vi "Begin.vi"(8 "error in":errorcluster) -> (0 "error out":errorcluster)   [LabVIEW 2019]
doc: "Called before other user functions, this VI is expected to open initial I/O refnums, load in file data, and do all program initialization. Notice that the <B>error out</B> terminal is simply used for data flow. Wiring it to other structures or subVIs ensures that this VI runs first."
uses:
  <vilib>/Rock Robotics/WPI/DriverStation/WPI_DriverStationRobotMode2.ctl
  <vilib>/Rock Robotics/WPI/Joystick/WPI_JoystickDeviceEnum.ctl
  <vilib>/Rock Robotics/WPI/ThirdParty/Phoenix-LabVIEW/Motor Controller/Controls/CTRE_Phoenix_MotorControl_NeutralMode.ctl
  <vilib>/Rock Robotics/WPI/Solenoid/WPI_SolenoidChannel.ctl
  <vilib>/Rock Robotics/SystemInterfaces/DIO/FPGA_DIOChannel.ctl
  Robot Global Data.vi
  <vilib>/Rock Robotics/WPI/Utilities/WPI_GetSetVariantRefNum.vi
  <vilib>/Rock Robotics/WPI/Solenoid/WPI_SolenoidOpenDouble.vi
  <vilib>/Rock Robotics/WPI/ThirdParty/REV Robotics/SPARK MAX/Typedef/Spark MAX Idle Mode.ctl
  <vilib>/Rock Robotics/WPI/ThirdParty/Phoenix-LabVIEW/Motor Controller/Controls/CTRE_Phoenix_MotorControl_SupplyCurrentLimitConfiguration.ctl
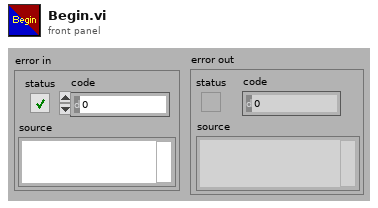
[diagram p1: front panel]
types:
  T1 = typedef "WPI_JoystickDeviceEnum.ctl" = enum16{"USB 0", "USB 1", "USB 2", "USB 3", "USB 4", "USB 5"}
  T2 = typedef "WPI_DriverStationRobotMode2.ctl" = enum16{"Autonomous Disabled", "Autonomous Enabled", "Teleop Disabled", "Teleop Enabled", "Disconnected", "Finish", "Test Disabled", "Test Enabled", "Emergency Stopped"}
  T3 = typedef "WPI_JoystickDevRef.ctl" = cluster{"Device":T1}
  T4 = typedef "Spark MAX Idle Mode.ctl" = enum16{"Coast", "Brake"}
  T5 = typedef "WPI_MotorControlDeviceRef.ctl" = cluster{"DeviceStatus":errorcluster, "Type":T6, "PWM":cluster{"PWM Channel":T7, "DeadBand":T8}, "CAN":cluster{"Device Number":u8, "SetOutput VI Ref":variant, "GetOutput VI Ref":variant, "Enable VI Ref":variant, "Disable VI Ref":variant, "Data":variant}, "Invert":bool, "DIO PWM":cluster{"PWM \"Enable\" Channel":T7, "DIOChannel":T9, "PWM Rate":dbl}}
  T6 = typedef "WPI_MotorControlType.ctl" = enum16{"PWM", "CAN", "DIO PWM"}
  T7 = typedef "FPGA_DIOPWMChannel.ctl" = enum8{"PWM 0", "PWM 1", "PWM 2", "PWM 3", "PWM 4", "PWM 5", "PWM 6", "PWM 7", "PWM 8", "PWM 9", "PWM MXP 0", "PWM MXP 1", "PWM MXP 2", "PWM MXP 3", "PWM MXP 4", "PWM MXP 5", "PWM MXP 6", "PWM MXP 7", "PWM MXP 8", "PWM MXP 9", "Invalid"}
  T8 = typedef "WPI_PWMDeadband.ctl" = cluster{"Name":string, "maxPositivePwm":i32, "minPositivePwm":i32, "centerPwm":i32, "maxNegativePwm":i32, "minNegativePwm":i32, "angularRange":u16}
  T9 = typedef "FPGA_DIOChannel.ctl" = enum8{"DIO 0", "DIO 1", "DIO 2", "DIO 3", "DIO 4", "DIO 5", "DIO 6", "DIO 7", "DIO 8", "DIO 9", "DIO MXP 0", "DIO MXP 1", "DIO MXP 2", "DIO MXP 3", "DIO MXP 4", "DIO MXP 5", "DIO MXP 6", "DIO MXP 7", "DIO MXP 8", "DIO MXP 9", "DIO MXP 10", "DIO MXP 11", "DIO MXP 12", "DIO MXP 13", "DIO MXP 14", "DIO MXP 15", "SPI Port CS1", "SPI Port CS2", "SPI Port CS3", "SPI Port MISO", "SPI Port MOSI", "Invalid"}
  T10 = typedef "CTRE_Phoenix_MotorControl_NeutralMode.ctl" = enum8{"EEPROMSetting", "Override to Coast", "Override to Brake"}
  T11 = typedef "CTRE_Phoenix_MotorControl_SupplyCurrentLimitConfiguration.ctl" = cluster{"Enable?":bool, "Current Limit":dbl, "Threshold Current":dbl, "Threshold Time":dbl}
  T12 = typedef "WPI_SolenoidChannel.ctl" = enum8{"Solenoid 0", "Solenoid 1", "Solenoid 2", "Solenoid 3", "Solenoid 4", "Solenoid 5", "Solenoid 6", "Solenoid 7", "Invalid"}
  T13 = typedef "WPI_CompressorDevRef.ctl" = cluster{"DevStatus":errorcluster, "Pneumatics Control Module":u8}
  T14 = typedef "WPI_SolenoidDevRef.ctl" = cluster{"DevStatus":errorcluster, "Pneumatics Control Module":u8, "Forward Solenoid Channel":T12, "Reverse Solenoid Channel":T12}
  T15 = typedef "WPI_DigitalInputDevRef.ctl" = cluster{"DevStatus":errorcluster, "DIO Channel":T9}
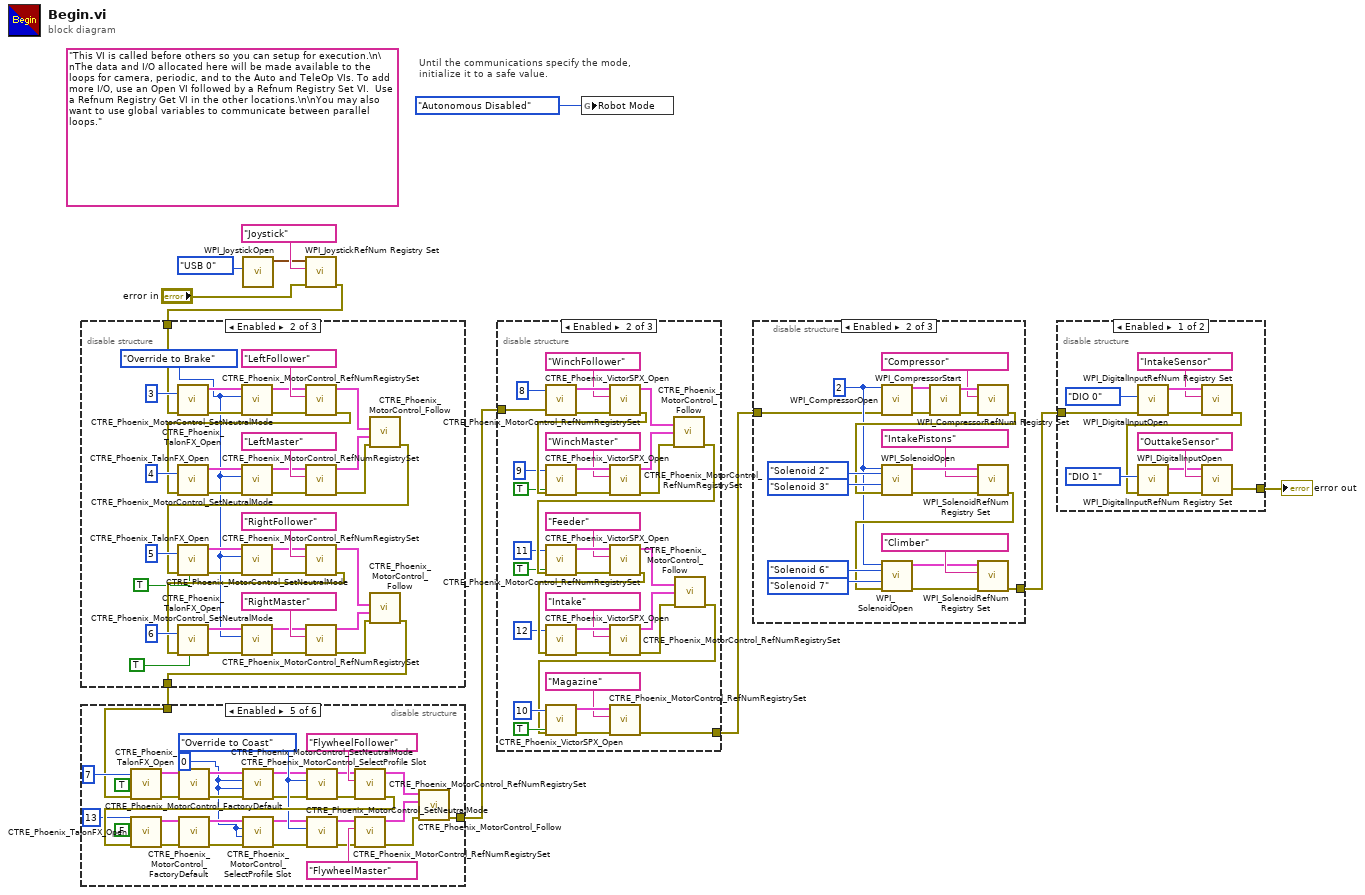
[diagram p0: block diagram]
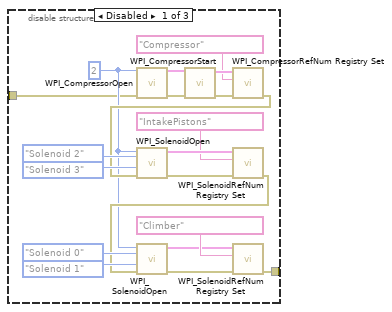
[diagram p3: hidden frame]
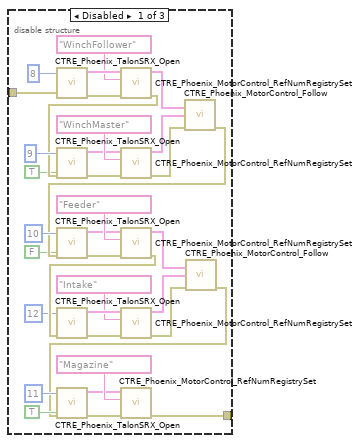
[diagram p5: hidden frame]
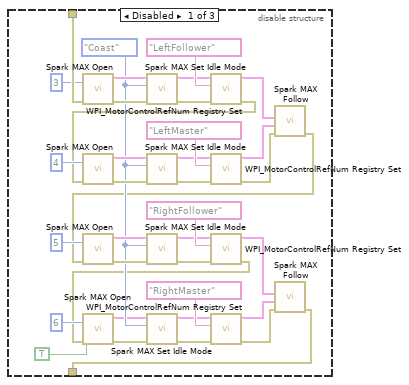
[diagram p7: hidden frame]
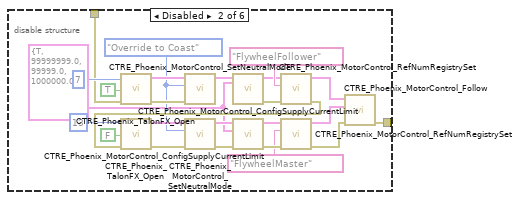
[diagram p10: hidden frame]
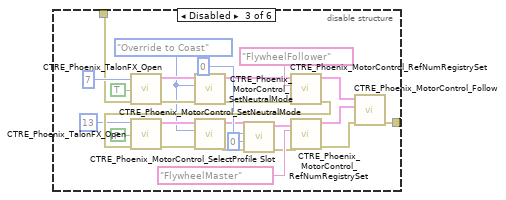
[diagram p11: hidden frame]
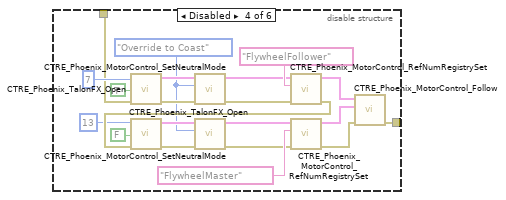
[diagram p12: hidden frame]
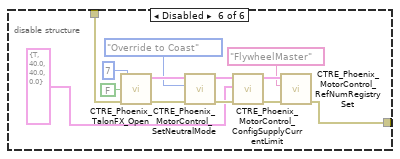
[diagram p13: hidden frame]
diagram:
  (unwired) "This VI is called before others so you can setup for execution.\n\nThe data and I/O allocated here will be made available to the loops for camera, periodic, and to the Auto and TeleOp VIs. To add more I/O, use an Open VI followed by a Refnum Registry Set VI.  Use a Refnum Registry Get VI in the other locations.\n\nYou may also want to use global variables to communicate between parallel loops."
  # "Until the communications specify the mode,\ninitialize it to a safe value."
  n1 = call <vilib>:"WPI_JoystickOpen.vi"("JoystickDevice"=WPI_JoystickDeviceEnum."USB 0") -> ("JoystickDevRef"=w9:T3)  [unwired: 10 in]
  n2 = call <vilib>:"WPI_JoystickRefNum Registry Set.vi"("error in (no error)"="error in", "refnum name"="Joystick", "JoystickDevRef"=w9) -> ("error out"=w7:errorcluster)  [unwired: 7 in, 1 out]
  n3 = disable-structure shown="Enabled" {
    disable-tunnel: w7 -> [w48 w52 w87]
    disable-tunnel: [w47 w51 w87] -> w5
    frame Disabled {
      w22 = Spark_MAX_Idle_Mode."Coast" ("Idle Mode")
      n4 = call <vilib>:"Spark MAX Open.vi"("error in (no error)"=w48, "Device Number"=u8 3) -> ("error out"=w33:errorcluster, "MotorControlDeviceRef"=w34:T5)  [unwired: 8 in]
      n5 = call <vilib>:"Spark MAX Set Idle Mode.vi"("error in (no error)"=w33, "Idle Mode"=w22, "MotorControlDeviceRef in"=w34) -> ("error out"=w31:errorcluster, "MotorControlDeviceRef out"=w32:T5)  [unwired: 7 in]
      n6 = call <vilib>:"WPI_MotorControlRefNum Registry Set.vi"("error in (no error)"=w31, "refnum name"="LeftFollower", "MotorControlDevRef"=w32) -> ("error out"=w17:errorcluster, "MotorControlDevRef"=w38:T5)  [unwired: 7 in]
      n7 = call <vilib>:"Spark MAX Open.vi"("error in (no error)"=w17, "Device Number"=u8 4) -> ("error out"=w29:errorcluster, "MotorControlDeviceRef"=w30:T5)  [unwired: 8 in]
      n8 = call <vilib>:"Spark MAX Set Idle Mode.vi"("error in (no error)"=w29, "Idle Mode"=w22, "MotorControlDeviceRef in"=w30) -> ("error out"=w27:errorcluster, "MotorControlDeviceRef out"=w28:T5)  [unwired: 7 in]
      n9 = call <vilib>:"WPI_MotorControlRefNum Registry Set.vi"("error in (no error)"=w27, "refnum name"="LeftMaster", "MotorControlDevRef"=w28) -> ("error out"=w16:errorcluster, "MotorControlDevRef"=w37:T5)  [unwired: 7 in]
      n10 = call <vilib>:"Spark MAX Follow.vi"("error in (no error)"=w16, "Master Controller"=w37, "MotorControlDeviceRef"=w38) -> ("error out"=w15:errorcluster)  [unwired: 7 in, 1 out]
      n11 = call <vilib>:"Spark MAX Open.vi"("error in (no error)"=w15, "Device Number"=u8 5) -> ("error out"=w25:errorcluster, "MotorControlDeviceRef"=w26:T5)  [unwired: 8 in]
      n12 = call <vilib>:"Spark MAX Set Idle Mode.vi"("error in (no error)"=w25, "Idle Mode"=w22, "MotorControlDeviceRef in"=w26) -> ("error out"=w23:errorcluster, "MotorControlDeviceRef out"=w24:T5)  [unwired: 7 in]
      n13 = call <vilib>:"WPI_MotorControlRefNum Registry Set.vi"("error in (no error)"=w23, "refnum name"="RightFollower", "MotorControlDevRef"=w24) -> ("error out"=w14:errorcluster, "MotorControlDevRef"=w36:T5)  [unwired: 7 in]
      n14 = call <vilib>:"Spark MAX Open.vi"("error in (no error)"=w14, "Invert"=TRUE, "Device Number"=u8 6) -> ("error out"=w20:errorcluster, "MotorControlDeviceRef"=w21:T5)  [unwired: 7 in]
      n15 = call <vilib>:"Spark MAX Set Idle Mode.vi"("error in (no error)"=w20, "Idle Mode"=w22, "MotorControlDeviceRef in"=w21) -> ("error out"=w18:errorcluster, "MotorControlDeviceRef out"=w19:T5)  [unwired: 7 in]
      n16 = call <vilib>:"WPI_MotorControlRefNum Registry Set.vi"("error in (no error)"=w18, "refnum name"="RightMaster", "MotorControlDevRef"=w19) -> ("error out"=w13:errorcluster, "MotorControlDevRef"=w35:T5)  [unwired: 7 in]
      n17 = call <vilib>:"Spark MAX Follow.vi"("error in (no error)"=w13, "Master Controller"=w35, "MotorControlDeviceRef"=w36) -> ("error out"=w47:errorcluster)  [unwired: 7 in, 1 out]
    }
    frame Enabled {
      w50 = CTRE_Phoenix_MotorControl_NeutralMode."Override to Brake" ("Motor Control Neutral Mode")
      n18 = call <vilib>:"CTRE_Phoenix_TalonFX_Open.vi"("error in"=w52, "Device Number"=u8 3) -> ("error out"=w73:errorcluster, "CAN Talon SRX Ref"=w74:T5)  [unwired: 8 in]
      n19 = call <vilib>:"CTRE_Phoenix_MotorControl_SetNeutralMode.vi"("error in (no error)"=w73, "Motor Control Neutral Mode"=w50, "PhoenixMotorControlDevRef"=w74) -> ("error out"=w71:errorcluster, "PhoenixMotorControlDevRef"=w72:T5)  [unwired: 7 in]
      n20 = call <vilib>:"CTRE_Phoenix_MotorControl_RefNumRegistrySet.vi"("error in (no error)"=w71, "refnum name"="LeftFollower", "PhoenixMotorControlDevRef"=w72) -> ("error out"=w58:errorcluster, "PhoenixMotorControlDevRef"=w78:T5)  [unwired: 7 in]
      n21 = call <vilib>:"CTRE_Phoenix_TalonFX_Open.vi"("error in"=w58, "Device Number"=u8 4) -> ("error out"=w69:errorcluster, "CAN Talon SRX Ref"=w70:T5)  [unwired: 8 in]
      n22 = call <vilib>:"CTRE_Phoenix_MotorControl_SetNeutralMode.vi"("error in (no error)"=w69, "Motor Control Neutral Mode"=w50, "PhoenixMotorControlDevRef"=w70) -> ("error out"=w67:errorcluster, "PhoenixMotorControlDevRef"=w68:T5)  [unwired: 7 in]
      n23 = call <vilib>:"CTRE_Phoenix_MotorControl_RefNumRegistrySet.vi"("error in (no error)"=w67, "refnum name"="LeftMaster", "PhoenixMotorControlDevRef"=w68) -> ("error out"=w57:errorcluster, "PhoenixMotorControlDevRef"=w77:T5)  [unwired: 7 in]
      n24 = call <vilib>:"CTRE_Phoenix_MotorControl_Follow.vi"("error in (no error)"=w57, "Master Controller to Follow"=w77, "PhoenixMotorControlDevRef"=w78) -> ("error out"=w56:errorcluster)  [unwired: 7 in, 1 out]
      n25 = call <vilib>:"CTRE_Phoenix_TalonFX_Open.vi"("Invert"=TRUE, "error in"=w56, "Device Number"=u8 5) -> ("error out"=w65:errorcluster, "CAN Talon SRX Ref"=w66:T5)  [unwired: 7 in]
      n26 = call <vilib>:"CTRE_Phoenix_MotorControl_SetNeutralMode.vi"("error in (no error)"=w65, "Motor Control Neutral Mode"=w50, "PhoenixMotorControlDevRef"=w66) -> ("error out"=w63:errorcluster, "PhoenixMotorControlDevRef"=w64:T5)  [unwired: 7 in]
      n27 = call <vilib>:"CTRE_Phoenix_MotorControl_RefNumRegistrySet.vi"("error in (no error)"=w63, "refnum name"="RightFollower", "PhoenixMotorControlDevRef"=w64) -> ("error out"=w55:errorcluster, "PhoenixMotorControlDevRef"=w76:T5)  [unwired: 7 in]
      n28 = call <vilib>:"CTRE_Phoenix_TalonFX_Open.vi"("Invert"=TRUE, "error in"=w55, "Device Number"=u8 6) -> ("error out"=w61:errorcluster, "CAN Talon SRX Ref"=w62:T5)  [unwired: 7 in]
      n29 = call <vilib>:"CTRE_Phoenix_MotorControl_SetNeutralMode.vi"("error in (no error)"=w61, "Motor Control Neutral Mode"=w50, "PhoenixMotorControlDevRef"=w62) -> ("error out"=w59:errorcluster, "PhoenixMotorControlDevRef"=w60:T5)  [unwired: 7 in]
      n30 = call <vilib>:"CTRE_Phoenix_MotorControl_RefNumRegistrySet.vi"("error in (no error)"=w59, "refnum name"="RightMaster", "PhoenixMotorControlDevRef"=w60) -> ("error out"=w54:errorcluster, "PhoenixMotorControlDevRef"=w75:T5)  [unwired: 7 in]
      n31 = call <vilib>:"CTRE_Phoenix_MotorControl_Follow.vi"("error in (no error)"=w54, "Master Controller to Follow"=w75, "PhoenixMotorControlDevRef"=w76) -> ("error out"=w51:errorcluster)  [unwired: 7 in, 1 out]
    }
    frame Disabled {
    }
  }
  n32 = disable-structure shown="Enabled" {
    disable-tunnel: w5 -> [w88 w109 w134 w155 w187 w193]
    disable-tunnel: [w88 w89 w122 w143 w177 w190] -> w4
    frame Disabled {
    }
    frame Disabled {
      w97 = T11 {"Enable?"=TRUE, "Current Limit"=99999999.0, "Threshold Current"=99999.0, "Threshold Time"=1000000.0} ("Supply Current Limit Configuration")
      w98 = CTRE_Phoenix_MotorControl_NeutralMode."Override to Coast" ("Motor Control Neutral Mode")
      n33 = call <vilib>:"CTRE_Phoenix_TalonFX_Open.vi"("Invert"=TRUE, "error in"=w109, "Device Number"=u8 7) -> ("error out"=w110:errorcluster, "CAN Talon SRX Ref"=w111:T5)  [unwired: 7 in]
      n34 = call <vilib>:"CTRE_Phoenix_MotorControl_SetNeutralMode.vi"("error in (no error)"=w110, "Motor Control Neutral Mode"=w98, "PhoenixMotorControlDevRef"=w111) -> ("PhoenixMotorControlDevRef"=w106:T5)  [unwired: 7 in, 1 out]
      n35 = call <vilib>:"CTRE_Phoenix_MotorControl_ConfigSupplyCurrentLimit.vi"("Supply Current Limit Configuration"=w97, "PhoenixMotorControlDevRef"=w106) -> ("error out"=w108:errorcluster, "PhoenixMotorControlDevRef"=w107:T5)  [unwired: 8 in]
      n36 = call <vilib>:"CTRE_Phoenix_MotorControl_RefNumRegistrySet.vi"("error in (no error)"=w108, "refnum name"="FlywheelFollower", "PhoenixMotorControlDevRef"=w107) -> ("error out"=w99:errorcluster, "PhoenixMotorControlDevRef"=w95:T5)  [unwired: 7 in]
      n37 = call <vilib>:"CTRE_Phoenix_TalonFX_Open.vi"("Invert"=FALSE, "error in"=w99, "Device Number"=u8 13) -> ("error out"=w104:errorcluster, "CAN Talon SRX Ref"=w105:T5)  [unwired: 7 in]
      n38 = call <vilib>:"CTRE_Phoenix_MotorControl_SetNeutralMode.vi"("error in (no error)"=w104, "Motor Control Neutral Mode"=w98, "PhoenixMotorControlDevRef"=w105) -> ("error out"=w100:errorcluster, "PhoenixMotorControlDevRef"=w101:T5)  [unwired: 7 in]
      n39 = call <vilib>:"CTRE_Phoenix_MotorControl_ConfigSupplyCurrentLimit.vi"("error in (no error)"=w100, "Supply Current Limit Configuration"=w97, "PhoenixMotorControlDevRef"=w101) -> ("error out"=w103:errorcluster, "PhoenixMotorControlDevRef"=w102:T5)  [unwired: 7 in]
      n40 = call <vilib>:"CTRE_Phoenix_MotorControl_RefNumRegistrySet.vi"("error in (no error)"=w103, "refnum name"="FlywheelMaster", "PhoenixMotorControlDevRef"=w102) -> ("error out"=w93:errorcluster, "PhoenixMotorControlDevRef"=w94:T5)  [unwired: 7 in]
      n41 = call <vilib>:"CTRE_Phoenix_MotorControl_Follow.vi"("error in (no error)"=w93, "Master Controller to Follow"=w94, "PhoenixMotorControlDevRef"=w95) -> ("error out"=w89:errorcluster)  [unwired: 7 in, 1 out]
    }
    frame Disabled {
      w130 = CTRE_Phoenix_MotorControl_NeutralMode."Override to Coast" ("Motor Control Neutral Mode")
      n42 = call <vilib>:"CTRE_Phoenix_TalonFX_Open.vi"("Invert"=TRUE, "error in"=w134, "Device Number"=u8 7) -> ("error out"=w135:errorcluster, "CAN Talon SRX Ref"=w136:T5)  [unwired: 7 in]
      n43 = call <vilib>:"CTRE_Phoenix_MotorControl_SetNeutralMode.vi"("error in (no error)"=w135, "Motor Control Neutral Mode"=w130, "PhoenixMotorControlDevRef"=w136) -> ("error out"=w115:errorcluster, "PhoenixMotorControlDevRef"=w116:T5)  [unwired: 7 in]
      n44 = call <vilib>:"CTRE_Phoenix_MotorControl_RefNumRegistrySet.vi"("error in (no error)"=w115, "refnum name"="FlywheelFollower", "PhoenixMotorControlDevRef"=w116) -> ("error out"=w131:errorcluster, "PhoenixMotorControlDevRef"=w128:T5)  [unwired: 7 in]
      n45 = call <vilib>:"CTRE_Phoenix_TalonFX_Open.vi"("Invert"=FALSE, "error in"=w131, "Device Number"=u8 13) -> ("error out"=w132:errorcluster, "CAN Talon SRX Ref"=w133:T5)  [unwired: 7 in]
      n46 = call <vilib>:"CTRE_Phoenix_MotorControl_SetNeutralMode.vi"("error in (no error)"=w132, "Motor Control Neutral Mode"=w130, "PhoenixMotorControlDevRef"=w133) -> ("error out"=w117:errorcluster, "PhoenixMotorControlDevRef"=w118:T5)  [unwired: 7 in]
      n47 = call <vilib>:"CTRE_Phoenix_MotorControl_SelectProfile Slot.vi"("error in (no error)"=w117, "pidLoopIdx"=0, "slotIdx"=0, "PhoenixMotorControlDevRef"=w118) -> ("error out"=w120:errorcluster, "PhoenixMotorControlDevRef"=w121:T5)  [unwired: 6 in]
      n48 = call <vilib>:"CTRE_Phoenix_MotorControl_RefNumRegistrySet.vi"("error in (no error)"=w120, "refnum name"="FlywheelMaster", "PhoenixMotorControlDevRef"=w121) -> ("error out"=w126:errorcluster, "PhoenixMotorControlDevRef"=w127:T5)  [unwired: 7 in]
      n49 = call <vilib>:"CTRE_Phoenix_MotorControl_Follow.vi"("error in (no error)"=w126, "Master Controller to Follow"=w127, "PhoenixMotorControlDevRef"=w128) -> ("error out"=w122:errorcluster)  [unwired: 7 in, 1 out]
    }
    frame Disabled {
      w151 = CTRE_Phoenix_MotorControl_NeutralMode."Override to Coast" ("Motor Control Neutral Mode")
      n50 = call <vilib>:"CTRE_Phoenix_TalonFX_Open.vi"("Invert"=TRUE, "error in"=w155, "Device Number"=u8 7) -> ("error out"=w156:errorcluster, "CAN Talon SRX Ref"=w157:T5)  [unwired: 7 in]
      n51 = call <vilib>:"CTRE_Phoenix_MotorControl_SetNeutralMode.vi"("error in (no error)"=w156, "Motor Control Neutral Mode"=w151, "PhoenixMotorControlDevRef"=w157) -> ("error out"=w142:errorcluster, "PhoenixMotorControlDevRef"=w141:T5)  [unwired: 7 in]
      n52 = call <vilib>:"CTRE_Phoenix_MotorControl_RefNumRegistrySet.vi"("error in (no error)"=w142, "refnum name"="FlywheelFollower", "PhoenixMotorControlDevRef"=w141) -> ("error out"=w152:errorcluster, "PhoenixMotorControlDevRef"=w149:T5)  [unwired: 7 in]
      n53 = call <vilib>:"CTRE_Phoenix_TalonFX_Open.vi"("Invert"=FALSE, "error in"=w152, "Device Number"=u8 13) -> ("error out"=w153:errorcluster, "CAN Talon SRX Ref"=w154:T5)  [unwired: 7 in]
      n54 = call <vilib>:"CTRE_Phoenix_MotorControl_SetNeutralMode.vi"("error in (no error)"=w153, "Motor Control Neutral Mode"=w151, "PhoenixMotorControlDevRef"=w154) -> ("error out"=w139:errorcluster, "PhoenixMotorControlDevRef"=w140:T5)  [unwired: 7 in]
      n55 = call <vilib>:"CTRE_Phoenix_MotorControl_RefNumRegistrySet.vi"("error in (no error)"=w139, "refnum name"="FlywheelMaster", "PhoenixMotorControlDevRef"=w140) -> ("error out"=w147:errorcluster, "PhoenixMotorControlDevRef"=w148:T5)  [unwired: 7 in]
      n56 = call <vilib>:"CTRE_Phoenix_MotorControl_Follow.vi"("error in (no error)"=w147, "Master Controller to Follow"=w148, "PhoenixMotorControlDevRef"=w149) -> ("error out"=w143:errorcluster)  [unwired: 7 in, 1 out]
    }
    frame Enabled {
      w164 = 0 ("slotIdx")
      w185 = CTRE_Phoenix_MotorControl_NeutralMode."Override to Coast" ("Motor Control Neutral Mode")
      n57 = call <vilib>:"CTRE_Phoenix_TalonFX_Open.vi"("Invert"=TRUE, "error in"=w187, "Device Number"=u8 7) -> ("error out"=w169:errorcluster, "CAN Talon SRX Ref"=w170:T5)  [unwired: 7 in]
      n58 = call <vilib>:"CTRE_Phoenix_MotorControl_FactoryDefault.vi"("error in"=w169, "PhoenixMotorControlDevRef"=w170) -> ("error out"=w168:errorcluster, "PhoenixMotorControlDevRef"=w167:T5)  [unwired: 8 in]
      n59 = call <vilib>:"CTRE_Phoenix_MotorControl_SelectProfile Slot.vi"("error in (no error)"=w168, "pidLoopIdx"=w164, "slotIdx"=w164, "PhoenixMotorControlDevRef"=w167) -> ("error out"=w162:errorcluster, "PhoenixMotorControlDevRef"=w163:T5)  [unwired: 6 in]
      n60 = call <vilib>:"CTRE_Phoenix_MotorControl_SetNeutralMode.vi"("error in (no error)"=w162, "Motor Control Neutral Mode"=w185, "PhoenixMotorControlDevRef"=w163) -> ("error out"=w175:errorcluster, "PhoenixMotorControlDevRef"=w176:T5)  [unwired: 7 in]
      n61 = call <vilib>:"CTRE_Phoenix_MotorControl_RefNumRegistrySet.vi"("error in (no error)"=w175, "refnum name"="FlywheelFollower", "PhoenixMotorControlDevRef"=w176) -> ("error out"=w186:errorcluster, "PhoenixMotorControlDevRef"=w183:T5)  [unwired: 7 in]
      n62 = call <vilib>:"CTRE_Phoenix_TalonFX_Open.vi"("Invert"=FALSE, "error in"=w186, "Device Number"=u8 13) -> ("error out"=w171:errorcluster, "CAN Talon SRX Ref"=w172:T5)  [unwired: 7 in]
      n63 = call <vilib>:"CTRE_Phoenix_MotorControl_FactoryDefault.vi"("error in"=w171, "PhoenixMotorControlDevRef"=w172) -> ("error out"=w165:errorcluster, "PhoenixMotorControlDevRef"=w166:T5)  [unwired: 8 in]
      n64 = call <vilib>:"CTRE_Phoenix_MotorControl_SelectProfile Slot.vi"("error in (no error)"=w165, "pidLoopIdx"=w164, "slotIdx"=w164, "PhoenixMotorControlDevRef"=w166) -> ("error out"=w160:errorcluster, "PhoenixMotorControlDevRef"=w161:T5)  [unwired: 6 in]
      n65 = call <vilib>:"CTRE_Phoenix_MotorControl_SetNeutralMode.vi"("error in (no error)"=w160, "Motor Control Neutral Mode"=w185, "PhoenixMotorControlDevRef"=w161) -> ("error out"=w173:errorcluster, "PhoenixMotorControlDevRef"=w174:T5)  [unwired: 7 in]
      n66 = call <vilib>:"CTRE_Phoenix_MotorControl_RefNumRegistrySet.vi"("error in (no error)"=w173, "refnum name"="FlywheelMaster", "PhoenixMotorControlDevRef"=w174) -> ("error out"=w181:errorcluster, "PhoenixMotorControlDevRef"=w182:T5)  [unwired: 7 in]
      n67 = call <vilib>:"CTRE_Phoenix_MotorControl_Follow.vi"("error in (no error)"=w181, "Master Controller to Follow"=w182, "PhoenixMotorControlDevRef"=w183) -> ("error out"=w177:errorcluster)  [unwired: 7 in, 1 out]
    }
    frame Disabled {
      n68 = call <vilib>:"CTRE_Phoenix_TalonFX_Open.vi"("Invert"=FALSE, "error in"=w193, "Device Number"=u8 7) -> ("error out"=w199:errorcluster, "CAN Talon SRX Ref"=w198:T5)  [unwired: 7 in]
      n69 = call <vilib>:"CTRE_Phoenix_MotorControl_SetNeutralMode.vi"("error in (no error)"=w199, "Motor Control Neutral Mode"=CTRE_Phoenix_MotorControl_NeutralMode."Override to Coast", "PhoenixMotorControlDevRef"=w198) -> ("error out"=w192:errorcluster, "PhoenixMotorControlDevRef"=w202:T5)  [unwired: 7 in]
      n70 = call <vilib>:"CTRE_Phoenix_MotorControl_ConfigSupplyCurrentLimit.vi"("error in (no error)"=w192, "Supply Current Limit Configuration"=T11 {"Enable?"=TRUE, "Current Limit"=40.0, "Threshold Current"=40.0, "Threshold Time"=0.0}, "PhoenixMotorControlDevRef"=w202) -> ("error out"=w200:errorcluster, "PhoenixMotorControlDevRef"=w201:T5)  [unwired: 7 in]
      n71 = call <vilib>:"CTRE_Phoenix_MotorControl_RefNumRegistrySet.vi"("error in (no error)"=w200, "refnum name"="FlywheelMaster", "PhoenixMotorControlDevRef"=w201) -> ("error out"=w190:errorcluster)  [unwired: 7 in, 1 out]
    }
  }
  n72 = disable-structure shown="Enabled" {
    disable-tunnel: w4 -> [w208 w243 w273]
    disable-tunnel: [w207 w242 w273] -> w3
    frame Disabled {
      n73 = call <vilib>:"CTRE_Phoenix_TalonSRX_Open.vi"("error in"=w208, "Device Number"=u8 8) -> ("error out"=w220:errorcluster, "CAN Talon SRX Ref"=w221:T5)  [unwired: 8 in]
      n74 = call <vilib>:"CTRE_Phoenix_MotorControl_RefNumRegistrySet.vi"("error in (no error)"=w220, "refnum name"="WinchFollower", "PhoenixMotorControlDevRef"=w221) -> ("error out"=w213:errorcluster, "PhoenixMotorControlDevRef"=w209:T5)  [unwired: 7 in]
      n75 = call <vilib>:"CTRE_Phoenix_TalonSRX_Open.vi"("Invert"=TRUE, "error in"=w213, "Device Number"=u8 9) -> ("error out"=w215:errorcluster, "CAN Talon SRX Ref"=w214:T5)  [unwired: 7 in]
      n76 = call <vilib>:"CTRE_Phoenix_MotorControl_RefNumRegistrySet.vi"("error in (no error)"=w215, "refnum name"="WinchMaster", "PhoenixMotorControlDevRef"=w214) -> ("error out"=w211:errorcluster, "PhoenixMotorControlDevRef"=w210:T5)  [unwired: 7 in]
      n77 = call <vilib>:"CTRE_Phoenix_MotorControl_Follow.vi"("error in (no error)"=w211, "Master Controller to Follow"=w210, "PhoenixMotorControlDevRef"=w209) -> ("error out"=w224:errorcluster)  [unwired: 7 in, 1 out]
      n78 = call <vilib>:"CTRE_Phoenix_TalonSRX_Open.vi"("Invert"=FALSE, "error in"=w224, "Device Number"=u8 10) -> ("error out"=w230:errorcluster, "CAN Talon SRX Ref"=w229:T5)  [unwired: 7 in]
      n79 = call <vilib>:"CTRE_Phoenix_MotorControl_RefNumRegistrySet.vi"("error in (no error)"=w230, "refnum name"="Feeder", "PhoenixMotorControlDevRef"=w229) -> ("error out"=w237:errorcluster, "PhoenixMotorControlDevRef"=w206:T5)  [unwired: 7 in]
      n80 = call <vilib>:"CTRE_Phoenix_TalonSRX_Open.vi"("error in"=w237, "Device Number"=u8 12) -> ("error out"=w235:errorcluster, "CAN Talon SRX Ref"=w236:T5)  [unwired: 8 in]
      n81 = call <vilib>:"CTRE_Phoenix_MotorControl_RefNumRegistrySet.vi"("error in (no error)"=w235, "refnum name"="Intake", "PhoenixMotorControlDevRef"=w236) -> ("error out"=w204:errorcluster, "PhoenixMotorControlDevRef"=w205:T5)  [unwired: 7 in]
      n82 = call <vilib>:"CTRE_Phoenix_MotorControl_Follow.vi"("error in (no error)"=w204, "Master Controller to Follow"=w205, "PhoenixMotorControlDevRef"=w206) -> ("error out"=w203:errorcluster)  [unwired: 7 in, 1 out]
      n83 = call <vilib>:"CTRE_Phoenix_TalonSRX_Open.vi"("Invert"=TRUE, "error in"=w203, "Device Number"=u8 11) -> ("error out"=w226:errorcluster, "CAN Talon SRX Ref"=w225:T5)  [unwired: 7 in]
      n84 = call <vilib>:"CTRE_Phoenix_MotorControl_RefNumRegistrySet.vi"("error in (no error)"=w226, "refnum name"="Magazine", "PhoenixMotorControlDevRef"=w225) -> ("error out"=w207:errorcluster)  [unwired: 7 in, 1 out]
    }
    frame Enabled {
      n85 = call <vilib>:"CTRE_Phoenix_VictorSPX_Open.vi"("error in"=w243, "Device Number"=u8 8) -> ("error out"=w266:errorcluster, "CAN Talon SRX Ref"=w265:T5)  [unwired: 8 in]
      n86 = call <vilib>:"CTRE_Phoenix_MotorControl_RefNumRegistrySet.vi"("error in (no error)"=w266, "refnum name"="WinchFollower", "PhoenixMotorControlDevRef"=w265) -> ("error out"=w269:errorcluster, "PhoenixMotorControlDevRef"=w272:T5)  [unwired: 7 in]
      n87 = call <vilib>:"CTRE_Phoenix_VictorSPX_Open.vi"("Invert"=TRUE, "error in"=w269, "Device Number"=u8 9) -> ("error out"=w267:errorcluster, "CAN Talon SRX Ref"=w268:T5)  [unwired: 7 in]
      n88 = call <vilib>:"CTRE_Phoenix_MotorControl_RefNumRegistrySet.vi"("error in (no error)"=w267, "refnum name"="WinchMaster", "PhoenixMotorControlDevRef"=w268) -> ("error out"=w270:errorcluster, "PhoenixMotorControlDevRef"=w271:T5)  [unwired: 7 in]
      n89 = call <vilib>:"CTRE_Phoenix_MotorControl_Follow.vi"("error in (no error)"=w270, "Master Controller to Follow"=w271, "PhoenixMotorControlDevRef"=w272) -> ("error out"=w264:errorcluster)  [unwired: 7 in, 1 out]
      n90 = call <vilib>:"CTRE_Phoenix_VictorSPX_Open.vi"("Invert"=TRUE, "error in"=w264, "Device Number"=u8 11) -> ("error out"=w260:errorcluster, "CAN Talon SRX Ref"=w261:T5)  [unwired: 7 in]
      n91 = call <vilib>:"CTRE_Phoenix_MotorControl_RefNumRegistrySet.vi"("error in (no error)"=w260, "refnum name"="Feeder", "PhoenixMotorControlDevRef"=w261) -> ("error out"=w257:errorcluster, "PhoenixMotorControlDevRef"=w241:T5)  [unwired: 7 in]
      n92 = call <vilib>:"CTRE_Phoenix_VictorSPX_Open.vi"("error in"=w257, "Device Number"=u8 12) -> ("error out"=w259:errorcluster, "CAN Talon SRX Ref"=w258:T5)  [unwired: 8 in]
      n93 = call <vilib>:"CTRE_Phoenix_MotorControl_RefNumRegistrySet.vi"("error in (no error)"=w259, "refnum name"="Intake", "PhoenixMotorControlDevRef"=w258) -> ("error out"=w239:errorcluster, "PhoenixMotorControlDevRef"=w240:T5)  [unwired: 7 in]
      n94 = call <vilib>:"CTRE_Phoenix_MotorControl_Follow.vi"("error in (no error)"=w239, "Master Controller to Follow"=w240, "PhoenixMotorControlDevRef"=w241) -> ("error out"=w238:errorcluster)  [unwired: 7 in, 1 out]
      n95 = call <vilib>:"CTRE_Phoenix_VictorSPX_Open.vi"("Invert"=TRUE, "error in"=w238, "Device Number"=u8 10) -> ("error out"=w262:errorcluster, "CAN Talon SRX Ref"=w263:T5)  [unwired: 7 in]
      n96 = call <vilib>:"CTRE_Phoenix_MotorControl_RefNumRegistrySet.vi"("error in (no error)"=w262, "refnum name"="Magazine", "PhoenixMotorControlDevRef"=w263) -> ("error out"=w242:errorcluster)  [unwired: 7 in, 1 out]
    }
    frame Disabled {
    }
  }
  n97 = global write "Robot Global Data.vi" "Robot Mode"(WPI_DriverStationRobotMode2."Autonomous Disabled" ("Robot Mode")) -> ()
  n98 = disable-structure shown="Enabled" {
    disable-tunnel: w3 -> [w275 w295 w314]
    disable-tunnel: [w274 w294 w314] -> w1
    frame Disabled {
      w276 = u8 2 ("Pneumatics Control Module (0)")
      n99 = call <vilib>:"WPI_CompressorOpen.vi"("Pneumatics Control Module (0)"=w276, "error in (no error)"=w275) -> ("CompressorDevRef"=w292:T13, "error out"=w293:errorcluster)  [unwired: 12 in]
      n100 = call <vilib>:"WPI_CompressorStart.vi"("error in (no error)"=w293, "CompressorDevRef"=w292) -> ("error out"=w291:errorcluster, "CompressorDevRef"=w290:T13)  [unwired: 8 in]
      n101 = call <vilib>:"WPI_CompressorRefNum Registry Set.vi"("error in (no error)"=w291, "refnum name"="Compressor", "CompressorDevRef"=w290) -> ("error out"=w278:errorcluster)  [unwired: 7 in, 1 out]
      n102 = call-poly <vilib>:"WPI_SolenoidOpen.vi"("error in (no error)"=w278, "Reverse Solenoid Channel"=WPI_SolenoidChannel."Solenoid 3", "Forward Solenoid Channel"=WPI_SolenoidChannel."Solenoid 2" ("Solenoid Channel"), "Pneumatics Control Module (0)"=w276) -> ("error out"=w287:errorcluster, "SolenoidDevRef"=w288:T14)  [unwired: 6 in]
      n103 = call <vilib>:"WPI_SolenoidRefNum Registry Set.vi"("error in (no error)"=w287, "refnum name"="IntakePistons", "SolenoidDevRef"=w288) -> ("error out"=w277:errorcluster)  [unwired: 7 in, 1 out]
      n104 = call-poly <vilib>:"WPI_SolenoidOpen.vi"("error in (no error)"=w277, "Reverse Solenoid Channel"=WPI_SolenoidChannel."Solenoid 1", "Forward Solenoid Channel"=WPI_SolenoidChannel."Solenoid 0" ("Solenoid Channel"), "Pneumatics Control Module (0)"=w276) -> ("error out"=w280:errorcluster, "SolenoidDevRef"=w279:T14)  [unwired: 6 in]
      n105 = call <vilib>:"WPI_SolenoidRefNum Registry Set.vi"("error in (no error)"=w280, "refnum name"="Climber", "SolenoidDevRef"=w279) -> ("error out"=w274:errorcluster)  [unwired: 7 in, 1 out]
    }
    frame Enabled {
      w296 = u8 2 ("Pneumatics Control Module (0)")
      n106 = call <vilib>:"WPI_CompressorOpen.vi"("Pneumatics Control Module (0)"=w296, "error in (no error)"=w295) -> ("CompressorDevRef"=w312:T13, "error out"=w313:errorcluster)  [unwired: 12 in]
      n107 = call <vilib>:"WPI_CompressorStart.vi"("error in (no error)"=w313, "CompressorDevRef"=w312) -> ("error out"=w311:errorcluster, "CompressorDevRef"=w310:T13)  [unwired: 8 in]
      n108 = call <vilib>:"WPI_CompressorRefNum Registry Set.vi"("error in (no error)"=w311, "refnum name"="Compressor", "CompressorDevRef"=w310) -> ("error out"=w298:errorcluster)  [unwired: 7 in, 1 out]
      n109 = call-poly <vilib>:"WPI_SolenoidOpen.vi"("error in (no error)"=w298, "Reverse Solenoid Channel"=WPI_SolenoidChannel."Solenoid 3", "Forward Solenoid Channel"=WPI_SolenoidChannel."Solenoid 2" ("Solenoid Channel"), "Pneumatics Control Module (0)"=w296) -> ("error out"=w307:errorcluster, "SolenoidDevRef"=w308:T14)  [unwired: 6 in]
      n110 = call <vilib>:"WPI_SolenoidRefNum Registry Set.vi"("error in (no error)"=w307, "refnum name"="IntakePistons", "SolenoidDevRef"=w308) -> ("error out"=w297:errorcluster)  [unwired: 7 in, 1 out]
      n111 = call-poly <vilib>:"WPI_SolenoidOpen.vi"("error in (no error)"=w297, "Reverse Solenoid Channel"=WPI_SolenoidChannel."Solenoid 7", "Forward Solenoid Channel"=WPI_SolenoidChannel."Solenoid 6" ("Solenoid Channel"), "Pneumatics Control Module (0)"=w296) -> ("error out"=w300:errorcluster, "SolenoidDevRef"=w299:T14)  [unwired: 6 in]
      n112 = call <vilib>:"WPI_SolenoidRefNum Registry Set.vi"("error in (no error)"=w300, "refnum name"="Climber", "SolenoidDevRef"=w299) -> ("error out"=w294:errorcluster)  [unwired: 7 in, 1 out]
    }
    frame Disabled {
    }
  }
  n113 = disable-structure shown="Enabled" {
    disable-tunnel: [w316 w326] -> w2
    disable-tunnel: w1 -> [w315 w326]
    frame Enabled {
      n114 = call <vilib>:"WPI_DigitalInputOpen.vi"("error in (no error)"=w315, "DIO Channel"=FPGA_DIOChannel."DIO 0") -> ("error out"=w324:errorcluster, "DigitalInputDevRef"=w325:T15)  [unwired: 8 in]
      n115 = call <vilib>:"WPI_DigitalInputRefNum Registry Set.vi"("error in (no error)"=w324, "refnum name"="IntakeSensor", "DigitalInputDevRef"=w325) -> ("error out"=w317:errorcluster)  [unwired: 7 in, 1 out]
      n116 = call <vilib>:"WPI_DigitalInputOpen.vi"("error in (no error)"=w317, "DIO Channel"=FPGA_DIOChannel."DIO 1") -> ("error out"=w319:errorcluster, "DigitalInputDevRef"=w318:T15)  [unwired: 8 in]
      n117 = call <vilib>:"WPI_DigitalInputRefNum Registry Set.vi"("error in (no error)"=w319, "refnum name"="OuttakeSensor", "DigitalInputDevRef"=w318) -> ("error out"=w316:errorcluster)  [unwired: 7 in, 1 out]
    }
    frame Disabled {
    }
  }
  "error out" <- w2
